vi "Main.vi"() -> ()   [LabVIEW 2021]
uses:
  System/bt_System.lvclass
  Support/Nodes/abs_Node/Status.ctl
  <vilib>/TSA/Event Log/Event_TextLog/Event_TextLog.lvclass/Event_TextLog.ctl
  <vilib>/TSA/Event Log/Event_TextLog/Event_TextLog.lvclass
  Support/Nodes/abs_Node/bt_Node.lvclass
panel:
  out "Log Display":string
  in  "Stop":bool
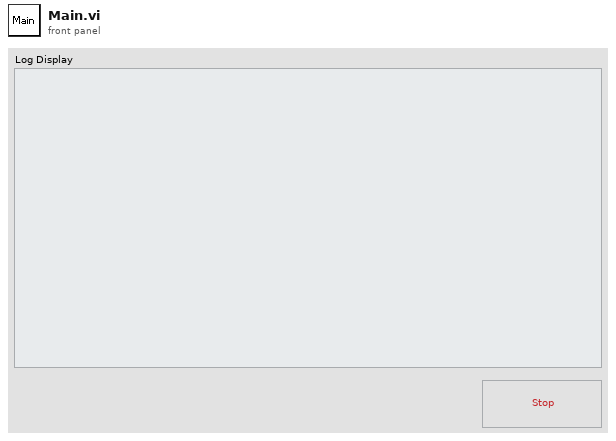
[diagram p1: front panel]
types:
  T1 = typedef "IO_Type.ctl" = cluster{"EventLog":refnum<class "Event_TextLog.lvclass">, "Blackboard":refnum<class "Blackboard.lvclass">}
  T2 = typedef "BT.lvlib/bt_Node.lvclass/Status.ctl" = enum16{"Success", "Failure", "Running"}
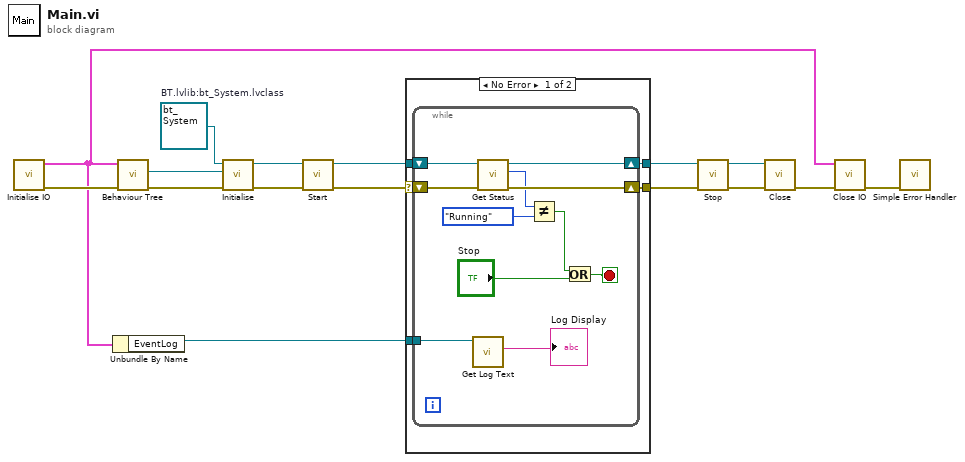
[diagram p0: block diagram]
diagram:
  w15 = refnum<class "bt_System.lvclass"> refnum  # BT.lvlib:bt_System.lvclass
  n1 = call "Initialise IO.vi"() -> ("error out"=w12:errorcluster, "IO"=w1:T1)  [unwired: 10 in]
  n2 = Unbundle By Name(w1) -> ("EventLog"=w16:refnum<class "Event_TextLog.lvclass">)
  n3 = call "Behaviour Tree.vi"("error in (no error)"=w12, "IO"=w1) -> ("error out"=w13:errorcluster, "Behaviour Tree"=w14:refnum<class "bt_Node.lvclass">)  [unwired: 8 in]
  n4 = call "Initialise.vi"("error in (no error)"=w13, "Behaviour Tree"=w14, "bt_System in"=w15) -> ("error out"=w10:errorcluster, "bt_System out"=w11:refnum<class "bt_System.lvclass">)  [unwired: 7 in]
  n5 = call "Start.vi"("error in (no error)"=w10, "bt_System in"=w11) -> ("error out"=w8:errorcluster, "bt_System out"=w9:refnum<class "bt_System.lvclass">)  [unwired: 8 in]
  n6 = case shown="No Error" w8 {
    selector: w8 -> [w20 w33]
    tunnel: w9 -> [w21 w34]
    tunnel: [w19 w34] -> w6
    tunnel: [w18 w33] -> w7
    tunnel: w16 -> [w17 _]
    frame No Error {
      n7 = while {
        shift-right: [w24] -> w19
        shift-left: w21 -> [w27]
        shift-right: [w25] -> w18
        shift-left: w20 -> [w26]
        tunnel: w17 -> [w28]
        stop <- w30 stop-if-true
        n8 = call <vilib>:"Get Log Text.vi"("Event_TextLog in"=w28) -> ("Log Message"=→"Log Display":string)  [unwired: 8 in, 2 out]
        n9 = call "Get Status.vi"("error in (no error)"=w26, "bt_System in"=w27) -> ("error out"=w25:errorcluster, "Status"=w22:T2, "bt_System out"=w24:refnum<class "bt_System.lvclass">)  [unwired: 7 in]
        n10 = Not Equal?(x=w22, y=Status."Running" ("Status")) -> (x != y?=w29:bool)
        n11 = Or(x=w29, y="Stop") -> (x .or. y?=w30:bool)
      }
    }
    frame Error {
    }
  }
  n12 = call "Stop.vi"("error in (no error)"=w7, "bt_System in"=w6) -> ("error out"=w4:errorcluster, "bt_System out"=w5:refnum<class "bt_System.lvclass">)  [unwired: 8 in]
  n13 = call-dynamic "Close.vi"("error in (no error)"=w4, "bt_System in"=w5) -> ("error out"=w3:errorcluster)  [unwired: 8 in, 1 out]
  n14 = call "Close IO.vi"("error in (no error)"=w3, "IO"=w1) -> ("error out"=w2:errorcluster)  [unwired: 9 in]
  n15 = call <vilib>:"Simple Error Handler.vi"("error in (no error)"=w2) -> ()  [unwired: 4 in, 5 out]
